vi "写配置.vi"(9 "adcgain":u8, 10 "LDOtrim":u8) -> (2 "result":bool)   [LabVIEW 2016]
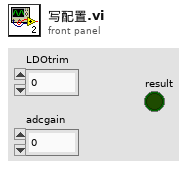
[diagram p1: front panel]
types:
  T1 = cluster{"byCmdType":u8, "bySubCmd":u8, "byPara":u8, "byAddr_h":u8, "byAddr_l":u8, "byAddr_ll":u8, "byLen_h":u8, "byLen_l":u8}
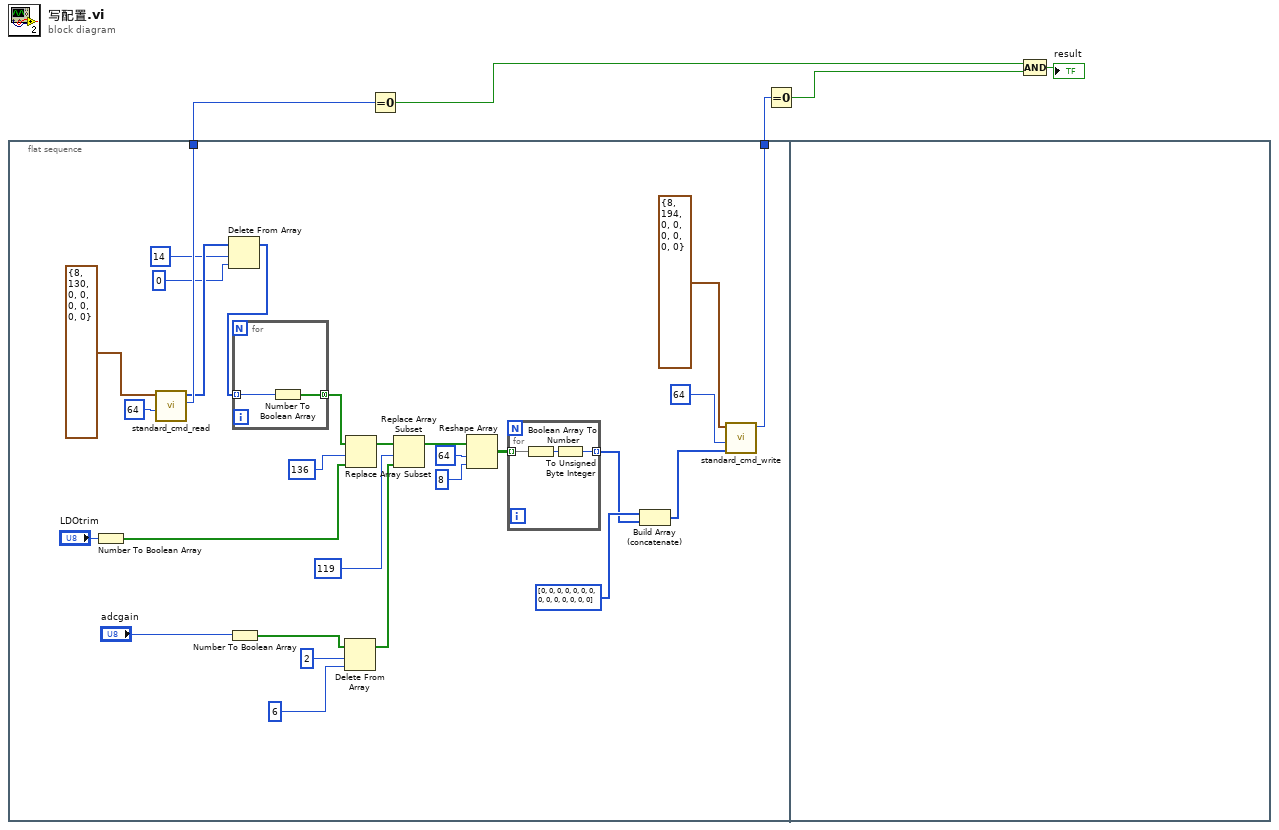
[diagram p0: block diagram]
diagram:
  n1 = flat-sequence {
    tunnel: [w22] -> w5
    tunnel: [w21] -> w4
    frame #0 {
      n2 = Number To Boolean Array(number="LDOtrim") -> (Boolean array=w17:bool[])
      n3 = call "standard_cmd_read.vi"("dwLen"=u32 64, "cmd_std_header_t"=T1 {"byCmdType"=8, "bySubCmd"=130, "byPara"=0, "byAddr_h"=0, "byAddr_l"=0, "byAddr_ll"=0, "byLen_h"=0, "byLen_l"=0}) -> ("return"=w22:i32, "data out"=w12:u8[])  [unwired: 7 in, 1 out]
      n4 = Delete From Array(array=w12, length=14, index=0) -> (array with subset deleted=w9:u8[])  [unwired: 1 out]
      n5 = Number To Boolean Array(number="adcgain") -> (Boolean array=w15:bool[])
      n6 = for {
        tunnel: w9 -> [w38] mode=indexing
        tunnel: [w37] -> w31 mode=concatenating
        n7 = Number To Boolean Array(number=w38) -> (Boolean array=w37:bool[])
      }
      n8 = Delete From Array(array=w15, length=2, index=6 ("length")) -> (array with subset deleted=w16:bool[])  [unwired: 1 out]
      n9 = Replace Array Subset(array=w31, new element=w17, index=136) -> (w30:bool[])
      n10 = Replace Array Subset(array=w30, new element=w16, index=119) -> (w27:bool[])
      n11 = Reshape Array(w27, 64 ("dimension size"), 8 ("dimension size")) -> (w25:bool[][])
      n12 = for {
        tunnel: w25 -> [w36] mode=indexing
        tunnel: [w34] -> w7 mode=indexing
        n13 = Boolean Array To Number(Boolean array=w36) -> (number=w35:u32)
        n14 = To Unsigned Byte Integer(number=w35) -> (unsigned 8bit integer=w34:u8)
      }
      n15 = Build Array (concatenate)(u8[] [0, 0, 0, 0, 0, 0, 0, 0, 0, 0, 0, 0, 0, 0], w7) -> (w6:u8[])
      n16 = call "standard_cmd_write.vi"("data"=w6, "dwLen"=64 ("dimension size"), "cmd_std_header_t"=T1 {"byCmdType"=8, "bySubCmd"=194, "byPara"=0, "byAddr_h"=0, "byAddr_l"=0, "byAddr_ll"=0, "byLen_h"=0, "byLen_l"=0}) -> ("return"=w21:i32)  [unwired: 7 in, 1 out]
    }
    frame #1 {
    }
  }
  n17 = Equal To 0?(x=w5) -> (x = 0?=w3:bool)
  n18 = Equal To 0?(x=w4) -> (x = 0?=w2:bool)
  n19 = Compound Arithmetic op=AND(w3, w2) -> (→"result":bool)
